vi "Access Privilege_VerifyInformation.vi"(8 "error in (no error)":errorcluster, 9 "Password":string, 10 "Name":string, 11 "Login Path":path=path "C:/Logindetails.dat") -> (0 "error out":errorcluster, 2 "Login Information":string[][](array[string]), 3 "Application Cluster":T1)   [LabVIEW 2023, in "GUI.lvlib"]
uses:
  GUI.lvlib
  Typedefs/Access Privilege_Account ManagerAppCluster.ctl
panel:
  in  "Application Cluster":T1
  out "Preference":string
  out "Numeric":i32
  out "Verified":bool
  out "Name confirmed":string
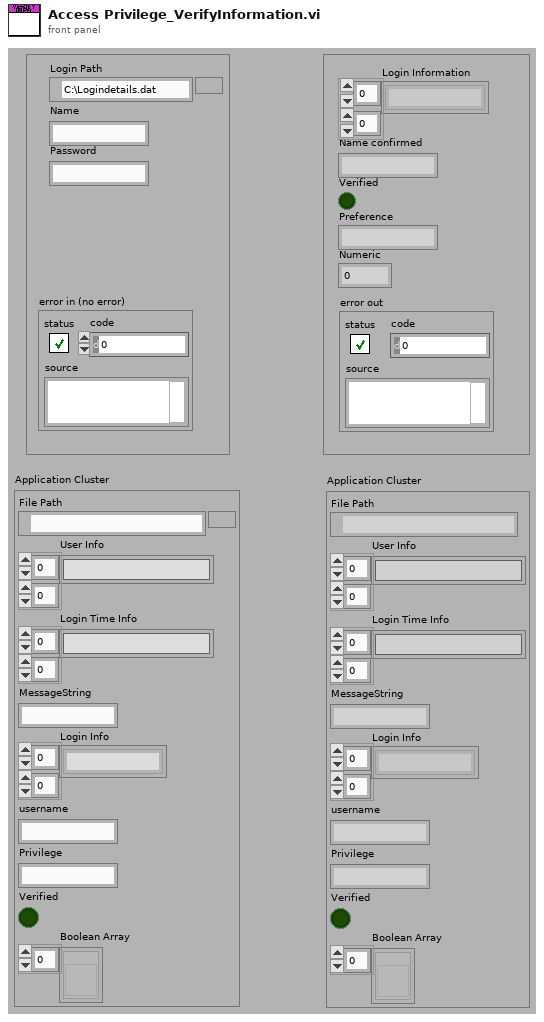
[diagram p1: front panel]
types:
  T1 = typedef "GUI.lvlib/Access Privilege_Account ManagerAppCluster.ctl" = cluster{"File Path":path, "User Info":string[][], "Login Time Info":string[][], "MessageString":string, "Login Info":string[][], "username":string, "Privilege":string, "Verified":bool, "Boolean Array":refnum<vi>[]}
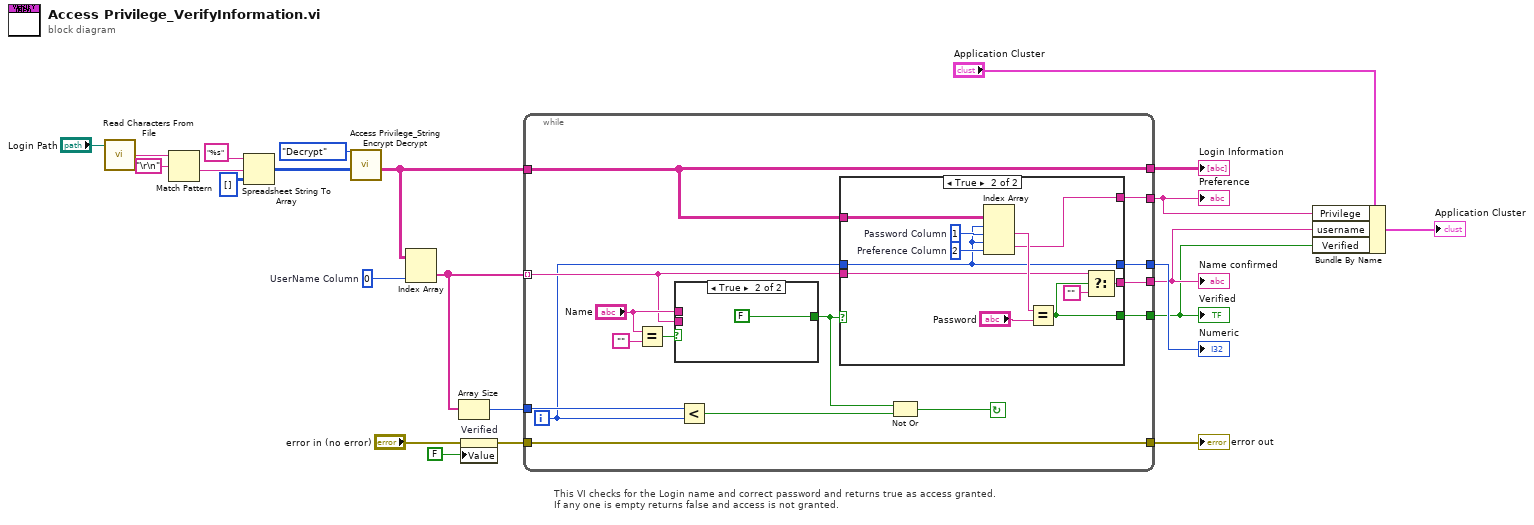
[diagram p0: block diagram]
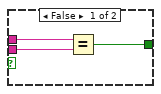
[diagram p2: hidden frame]
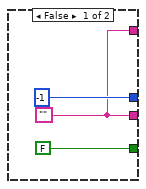
[diagram p3: hidden frame]
diagram:
  w23 = 0  # UserName Column
  # "This VI checks for the Login name and correct password and returns true as access granted.\nIf any one is empty returns false and access is not granted."
  n1 = call <vilib>:"Read Characters From File.vi"("file path (dialog if empty)"="Login Path") -> ("character string"=w12:string)  [unwired: 1 in, 7 out]
  n2 = Match Pattern(string=w12, regular expression="\r\n") -> (after substring=w10:string)  [unwired: 4 out]
  n3 = Spreadsheet String To Array(format string="%s", spreadsheet string=w10, array type (2D Dbl)=u8[][][] [] ("Encrypted Out")) -> (array=w13:u8[][][])  [unwired: 1 out]
  n4 = call "Access Privilege_String Encrypt Decrypt.vi"("Encrypted In"=w13, "Action"=enum16{"Encrypt", "Decrypt"}."Decrypt") -> ("Decrypted Out"=w15:string[][])  [unwired: 8 in, 1 out]
  n5 = Index Array(array=w15, index (col)=w23) -> (element=w22:string[])  [unwired: 1 in]
  n6 = Array Size(array=w22) -> (size(s)=w21:i32)
  n7 = property on="Verified" class="Bool (strict)"(error in="error in (no error)", "Value"=FALSE ("Verified")) -> (error out=w17:errorcluster)  [unwired: 1 in, 1 out]
  n8 = while {
    tunnel: w17 -> [w24]
    tunnel: [w32] -> w3
    tunnel: [w33] -> w20
    tunnel: [w34] -> w6
    tunnel: w22 -> [w27] mode=indexing
    tunnel: [w36] -> w4
    tunnel: w21 -> [w38]
    tunnel: w15 -> [w33]
    tunnel: [w25] -> w5
    tunnel: [w24] -> w7
    i -> [w26]
    stop <- w37 continue-if-true
    n9 = Equal?(x="Name", y="") -> (x = y?=w29:bool)
    n10 = case shown="True" w29 {
      tunnel: [w39 FALSE] -> w28
      tunnel: "Name" -> [w40 _]
      tunnel: w27 -> [w41 _]
      frame False {
        n11 = Equal?(x=w40, y=w41) -> (x = y?=w39:bool)
      }
      frame True {
      }
    }
    n12 = Less?(x=w38, y=w26) -> (x < y?=w35:bool)
    n13 = case shown="True" w28 {
      tunnel: w33 -> [_ w55]
      tunnel: w26 -> [_ w48]
      tunnel: [w43 w56] -> w36
      tunnel: [FALSE w51] -> w32
      tunnel: w27 -> [_ w52]
      tunnel: [-1 w48] -> w34
      tunnel: [w43 w46] -> w25
      frame False {
        w43 = ""
      }
      frame True {
        w49 = 2  # Preference Column
        w50 = 1  # Password Column
        n14 = Index Array(array=w55, index (row) #1=w48, index (col) #1=w50, index (row) #2=w48, index (col) #2=w49) -> (element #1=w54:string, element #2=w46:string)
        n15 = Equal?(x=w54, y="Password") -> (x = y?=w51:bool)
        n16 = Select(t=w52, s=w51, f="") -> (s? t:f=w56:string)
      }
    }
    n17 = Not Or(1:w35, 2:w28) -> (0:w37:bool)
  }
  "Name confirmed" <- w4
  "Verified" <- w3
  "Numeric" <- w6
  "Login Information" <- w20
  "Preference" <- w5
  "error out" <- w7
  n18 = Bundle By Name(cluster="Application Cluster", "Privilege"=w5, "username"=w4, "Verified"=w3) -> (→"Application Cluster":T1)
